vi "Create Submission.vi"(8 "error in (no error)":errorcluster, 9 "Challenge":refnum<class "Challenge.lvclass">, 10 "User":refnum<class "SOL User.lvclass">, 11 "Submission DB in":refnum<class "Submission DB.lvclass">) -> (0 "error out":errorcluster, 2 "Submission":refnum<class "Submission.lvclass">, 3 "Submission DB out":refnum<class "Submission DB.lvclass">)   [LabVIEW 2020, in "Summer of LabVIEW.lvlib" / "Submission DB.lvclass"]
uses:
  Submission DB.lvclass
  Submission DB.lvclass/Submission DB.ctl
  SOL User/SOL User.lvclass
  Challenge/Challenge.lvclass
  SQLite/SQLite.lvclass
  <vilib>/drjdpowell/SQLite Library/SQL Connection/Connection.lvclass
  <vilib>/IlluminatedG/lv-web-crypto/lv-json/JSON/JSON.lvlib
  <vilib>/drjdpowell/SQLite Library/SQL Statement/SQL Statement.lvclass
  SoL Scoring/Score Entry.ctl
  SoL Scoring/SoL Scoring.lvlib
  SoL Scoring/Score.ctl
  Submission/Submission Data.ctl
  Submission/Submission.lvclass
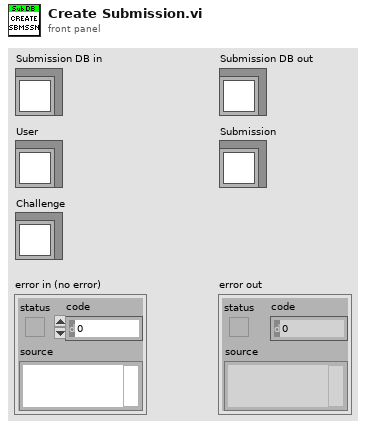
[diagram p1: front panel]
types:
  T1 = typedef "Summer of LabVIEW.lvlib/Submission.lvclass/Submission Data.ctl" = cluster{"ID":i64, "User ID":i64, "Challenge ID":i64, "Submitted":timestamp, "Score":T2, "Tested":bool, "Test Timestamp":timestamp, "Test Summary":string, "Approved for Test":bool, "Approver ID":i64}
  T2 = typedef "SoL Scoring.lvlib/Score.ctl" = cluster{"Overall":dbl, "Categories":T3[]}
  T3 = typedef "SoL Scoring.lvlib/Score Entry.ctl" = cluster{"Category":string, "Value":dbl}
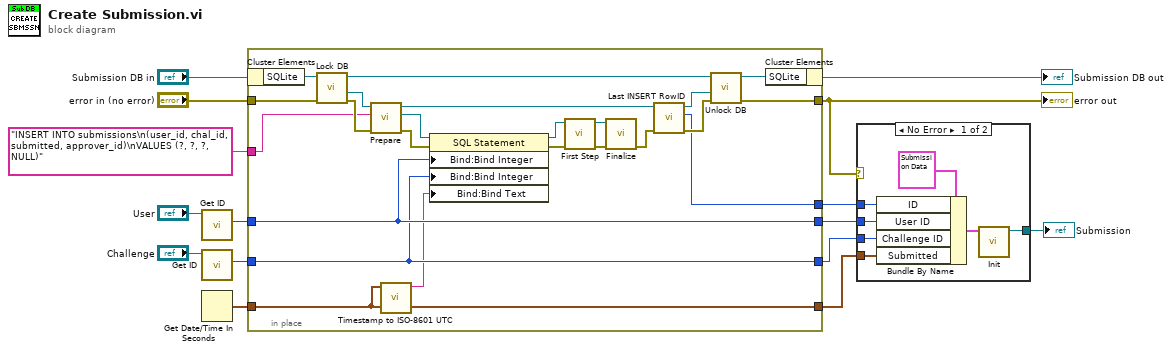
[diagram p0: block diagram]
diagram:
  n1 = call "Get ID.vi"("SOL User in"="User") -> ("ID"=w13:i64)  [unwired: 8 in, 2 out]
  n2 = call "Get ID.vi"("Challenge in"="Challenge") -> ("ID"=w12:i64)  [unwired: 9 in, 1 out]
  n3 = Get Date/Time In Seconds() -> (seconds since 1Jan1904=w8:timestamp)
  n4 = in-place {
    in-place-border: w13 -> [w19]
    in-place-border: w12 -> [w18]
    in-place-border: "error in (no error)" -> [w36]
    in-place-border: "INSERT INTO submissions\n(user_id, chal_id, submitted, approver_id)\nVALUES (?, ?, ?, NULL)" ("SQL") -> [w34]
    in-place-border: w8 -> [w16]
    in-place-border: [w21] -> w2
    in-place-border: [w20] -> w7
    in-place-border: [w19] -> w6
    in-place-border: [w18] -> w5
    in-place-border: [w16] -> w4
    n5 = in-place-cluster #1("Submission DB in") -> ("SQLite"=w37:refnum<class "SQLite.lvclass">)
    n6 = call "Lock DB.vi"("error in (no error)"=w36, "SQLite in"=w37) -> ("error out"=w38:errorcluster, "SQLite DB"=w35:refnum<class "Connection.lvclass">, "SQLite out"=w25:refnum<class "SQLite.lvclass">)  [unwired: 6 in, 1 out]
    n7 = call <vilib>:"Prepare.vi"("error in (no error)"=w38, "SQL"=w34, "SQLite Connection in"=w35) -> ("error out"=w32:errorcluster, "SQL Statement"=w33:refnum<class "SQL Statement.lvclass">, "SQLite Connection"=w26:refnum<class "Connection.lvclass">)  [unwired: 4 in, 2 out]
    n8 = call <vilib>:"Timestamp to ISO-8601 UTC.vi"("Time Stamp"=w16) -> ("ISO 8601 UTC"=w17:string)  [unwired: 10 in]
    n9 = property class="SQL Statement"(reference=w33, error in=w32, "Bind:Bind Integer"=w19, "Bind:Bind Integer"=w18, "Bind:Bind Text"=w17) -> (reference out=w29:refnum<class "SQL Statement.lvclass">, error out=w31:errorcluster)
    n10 = call <vilib>:"First Step.vi"("error in (no error)"=w31, "SQL Statement in"=w29) -> ("error out"=w30:errorcluster, "SQL Statement"=w28:refnum<class "SQL Statement.lvclass">)  [unwired: 7 in, 1 out]
    n11 = call <vilib>:"Finalize.vi"("error in (no error)"=w30, "SQL Statement in"=w28) -> ("error out"=w27:errorcluster)  [unwired: 9 in]
    n12 = call <vilib>:"Last INSERT RowID.vi"("error in (no error)"=w27, "SQLite Connection in"=w26) -> ("error out"=w23:errorcluster, "Last INSERT RowID"=w20:i64, "SQLite Connection"=w24:refnum<class "Connection.lvclass">)  [unwired: 7 in]
    n13 = call "Unlock DB.vi"("error in (no error)"=w23, "SQLite DB"=w24, "SQLite in"=w25) -> ("error out"=w21:errorcluster, "SQLite out"=w22:refnum<class "SQLite.lvclass">)  [unwired: 7 in]
    n14 = in-place-cluster #1("SQLite"=w22) -> (→"Submission DB out":refnum<class "Submission DB.lvclass">)
  }
  "error out" <- w2
  n15 = case shown="No Error" w2 {
    tunnel: w7 -> [w44 _]
    tunnel: w6 -> [w43 _]
    tunnel: w5 -> [w42 _]
    tunnel: w4 -> [w41 _]
    tunnel: [w39 _] -> w1
    frame No Error {
      n16 = Bundle By Name(cluster=T1 {"ID"=0, "User ID"=0, "Challenge ID"=0, "Submitted"=timestamp(0 s since 1904-01-01), "Score"={"Overall"=0.0, "Categories"=[]}, "Tested"=FALSE, "Test Timestamp"=timestamp(0 s since 1904-01-01), "Test Summary"="", "Approved for Test"=FALSE, "Approver ID"=0} ("Submission Data"), "ID"=w44, "User ID"=w43, "Challenge ID"=w42, "Submitted"=w41) -> (w40:T1)
      n17 = call "Init.vi"("Submission Data"=w40) -> ("Submission out"=w39:refnum<class "Submission.lvclass">)  [unwired: 9 in, 1 out]
    }
    frame Error {
    }
  }
  "Submission" <- w1
